vi "Format Gluing Config.vi"(4 "Active Paths":T2=[FALSE, FALSE, FALSE, FALSE], 6 "Glue Pathways":T3=[{"HDI Slot "=0, "Stamp Slot"=0, "Glue Slot"=0, "Weight Slot"=0, "BBM Slot"=0}, {"HDI Slot "=1, "Stamp Slot"=1, "Glue Slot"=1, "Weight Slot"=1, "BBM Slot"=1}, {"HDI Slot "=2, "Stamp Slot"=2, "Glue Slot"=2, "Weight Slot"=2, "BBM Slot"=2}, {"HDI Slot "=3, "Stamp Slot"=3, "Glue Slot"=3, "Weight Slot"=3, "BBM Slot"=3}] {"BBM Slot" items=["Slot 1", "Slot 2", "Slot 3", "Slot 4"]; "Weight Slot" items=["Slot 1", "Slot 2", "Slot 3", "Slot 4"]; "Glue Slot" items=["Slot 1", "Slot 2", "Slot 3", "Slot 4"]; "Stamp Slot" items=["Slot 1", "Slot 2", "Slot 3", "Slot 4"]; "HDI Slot" items=["Slot 1", "Slot 2", "Slot 3", "Slot 4"]}, 8 "error in":errorcluster, 9 "Chuck Module Used for BBM:":T1 items=["Chuck 1", "Chuck 2", "Chuck 3", "Chuck 4"], 10 "Worktable":refnum<class "WorkTable Class.lvclass">, 11 "Console Log in":refnum<class "Console Log.lvclass">) -> (0 "error out":errorcluster, 2 "Formatted Worktable Config":string, 3 "Console Log out":refnum<class "Console Log.lvclass">)   [LabVIEW 2011, in "Console Log.lvclass"]
uses:
  Console Log.lvclass
  Shared Components/WorkTable Class/WorkTable Class.lvclass
  Gluing Application/UI typedefs/Glue Paths.ctl
  Gluing Application/UI typedefs/Glue Path.ctl
  Gluing Application/UI typedefs/Active Paths.ctl
  Gluing Application/UI typedefs/BBM Chuck Used.ctl
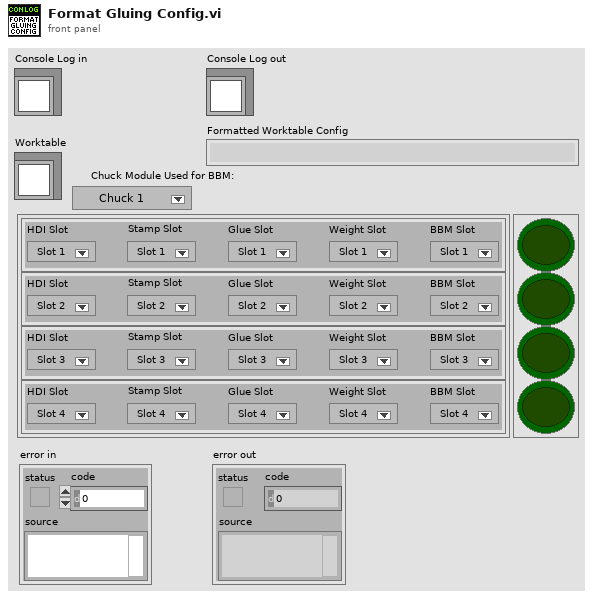
[diagram p1: front panel]
types:
  T1 = typedef "BBM Chuck Used.ctl" = i32
  T2 = typedef "Active Paths.ctl" = bool[]
  T3 = typedef "Glue Paths.ctl" = T4[]
  T4 = typedef "Glue Path.ctl" = cluster{"HDI Slot ":i32, "Stamp Slot":i32, "Glue Slot":i32, "Weight Slot":i32, "BBM Slot":i32}
  T5 = typedef "Worktable_Module Slot.ctl" = cluster{"Slot State":enum16{"Empty", "Bare HDI", "Unglued", "Stamped", "PartOnTop", "Weighted", "Unpotted", "Potted"}, "BBM Type":enum16{"None", "BBM", "GlassSlide"}, "HDI Type":enum16{"None", "HDI", "Polyimide"}, "Vacuum Channel":u8, "Location/Orientation BBM":T6, "Location/Orientation HDI":T6, "S/N":string}
  T6 = typedef "Position_Orientation.ctl" = cluster{"Center":refnum<class "Vec3d Class.lvclass">, "Orientation":refnum<class "Orient3d Class.lvclass">}
  T7 = typedef "Worktable_Stamps.ctl" = cluster{"Stamp Slots":T8[], "Vacuum Channel":i32}
  T8 = typedef "Worktable_Stamp.ctl" = cluster{"Stamp State":enum16{"Empty", "Populated", "Used"}, "Location/Orientation":T6, "Stamp Type":T9}
  T9 = typedef "Stamp Type.ctl" = enum16{"Stamp 1", "Stamp 2", "Stamp 3", "Stamp 4", "Stamp 5"}
  T10 = typedef "Worktable_Glue Reservoir.ctl" = cluster{"Glue Reservoir Slots":cluster{"Reservoir State":enum16{"Empty", "Full", "Used"}, "Center":refnum<class "Vec3d Class.lvclass">}[], "Vacuum Channel":i32}
  T11 = typedef "Worktable_Weights.ctl" = cluster{"Weight Slots":T12[], "Vacuum Channel":i32}
  T12 = typedef "Worktable_Weight.ctl" = cluster{"Weight State":enum16{"Empty", "Populated"}, "Weight Type":T13, "Location/Orientation":T6}
  T13 = typedef "Weight Type.ctl" = enum16{"Weight 1", "Weight 2", "Weight 3", "Weight 4", "Weight 5", "Weight 6", "Weight 7", "Weight 8"}
  T14 = cluster{"Reservoir State":enum16{"Empty", "Full", "Used"}, "Center":refnum<class "Vec3d Class.lvclass">}[]
  T15 = enum16{"Empty", "Bare HDI", "Unglued", "Stamped", "PartOnTop", "Weighted", "Unpotted", "Potted"}
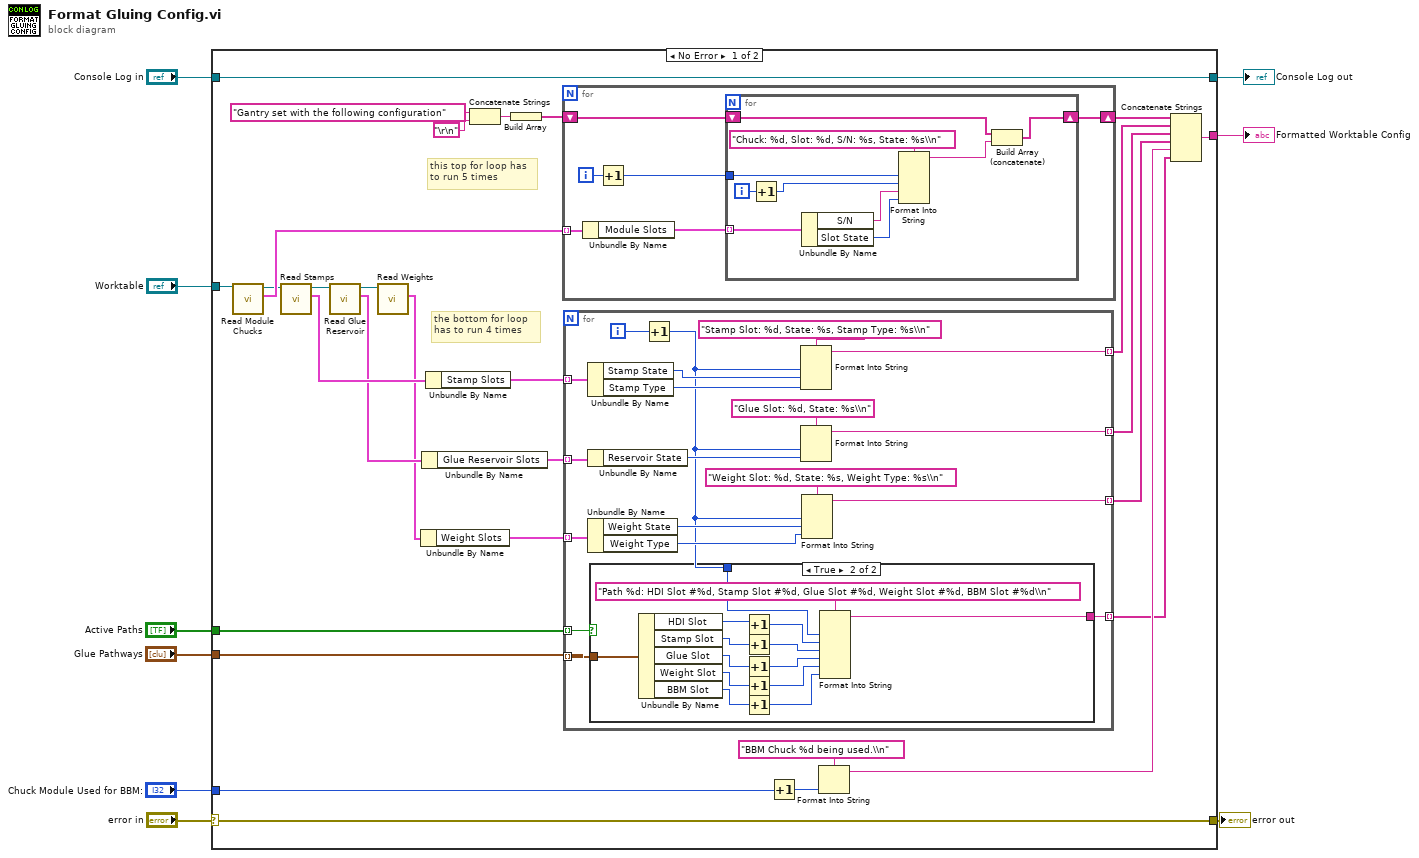
[diagram p0: block diagram]
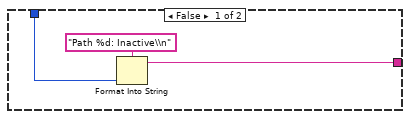
[diagram p2: hidden frame]
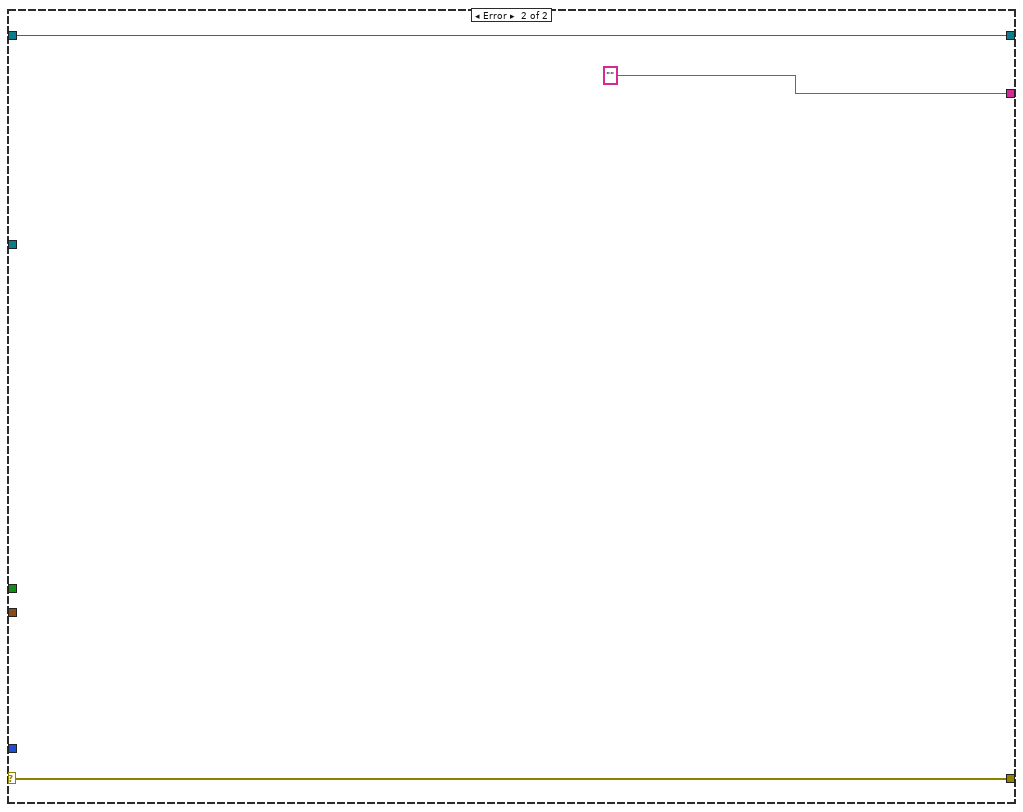
[diagram p3: hidden frame]
diagram:
  n1 = case shown="No Error" "error in" {
    selector: "error in" -> [w37 w93]
    tunnel: [w37 w93] -> w8
    tunnel: [w38 w92] -> w6
    tunnel: "Console Log in" -> [w38 w92]
    tunnel: "Worktable" -> [w29 _]
    tunnel: [w34 ""] -> w4
    tunnel: "Glue Pathways" -> [w22 _]
    tunnel: "Active Paths" -> [w21 _]
    tunnel: "Chuck Module Used for BBM:" -> [w10 _]
    frame No Error {
      # "this top for loop has\nto run 5 times"
      # "the bottom for loop\nhas to run 4 times"
      n2 = call-dynamic "Read Module Chucks.vi"("WorkTable in"=w29) -> ("Module Chucks"=w36:cluster{"Module Slots":T5[]}[], "WorkTable out"=w28:refnum<class "WorkTable Class.lvclass">)  [unwired: 8 in, 1 out]
      n3 = call-dynamic "Read Stamps.vi"("WorkTable Class in"=w28) -> ("Stamps"=w25:T7, "WorkTable Class out"=w27:refnum<class "WorkTable Class.lvclass">)  [unwired: 8 in, 1 out]
      n4 = call-dynamic "Read Glue Reservoir.vi"("WorkTable Class in"=w27) -> ("Glue Reservoir"=w24:T10, "WorkTable Class out"=w26:refnum<class "WorkTable Class.lvclass">)  [unwired: 8 in, 1 out]
      n5 = call-dynamic "Read Weights.vi"("WorkTable Class in"=w26) -> ("Weights"=w23:T11)  [unwired: 8 in, 2 out]
      n6 = Unbundle By Name(w23) -> ("Weight Slots"=w18:T12[])
      n7 = Unbundle By Name(w24) -> ("Glue Reservoir Slots"=w19:T14)
      n8 = Unbundle By Name(w25) -> ("Stamp Slots"=w20:T8[])
      n9 = Concatenate Strings("Gantry set with the following configuration", "\r\n") -> (w31:string)
      n10 = Build Array(w31) -> (w30:string[])
      n11 = for {
        tunnel: w36 -> [w80] mode=indexing
        shift-right: [w76] -> w35
        shift-left: w30 -> [w77]
        i -> [w78]
        n12 = Unbundle By Name(w80) -> ("Module Slots"=w79:T5[])
        n13 = Increment(x=w78) -> (x+1=w75:i32)
        n14 = for {
          tunnel: w79 -> [w90] mode=indexing
          tunnel: w75 -> [w88]
          shift-right: [w81] -> w76
          shift-left: w77 -> [w83]
          i -> [w89]
          n15 = Increment(x=w89) -> (x+1=w87:i32)
          n16 = Unbundle By Name(w90) -> ("S/N"=w85:string, "Slot State"=w84:T15)
          n17 = Format Into String(format string="Chuck: %d, Slot: %d, S/N: %s, State: %s\\n", w88, w87, w85, w84) -> (resulting string=w82:string)  [unwired: 2 in, 1 out]
          n18 = Build Array (concatenate)(w83, w82) -> (w81:string[])
        }
      }
      n19 = for {
        tunnel: w20 -> [w57] mode=indexing
        tunnel: w19 -> [w56] mode=indexing
        tunnel: w18 -> [w55] mode=indexing
        tunnel: [w46] -> w17 mode=indexing
        tunnel: [w45] -> w16 mode=indexing
        tunnel: [w44] -> w15 mode=indexing
        tunnel: w22 -> [w43] mode=indexing
        tunnel: w21 -> [w42] mode=indexing
        tunnel: [w41] -> w12 mode=indexing
        i -> [w40]
        n20 = Unbundle By Name(w57) -> ("Stamp State"=w53:enum16{"Empty", "Populated", "Used"}, "Stamp Type"=w52:T9)
        n21 = Unbundle By Name(w56) -> ("Reservoir State"=w50:enum16{"Empty", "Full", "Used"})
        n22 = Unbundle By Name(w55) -> ("Weight State"=w48:enum16{"Empty", "Populated"}, "Weight Type"=w47:T13)
        n23 = Increment(x=w40) -> (x+1=w39:i32)
        n24 = case shown="True" w42 {
          tunnel: w43 -> [_ w74]
          tunnel: w39 -> [w60 w73]
          tunnel: [w59 w71] -> w41
          frame False {
            n25 = Format Into String(format string="Path %d: Inactive\\n", w60) -> (resulting string=w59:string)  [unwired: 2 in, 1 out]
          }
          frame True {
            n26 = Unbundle By Name(w74) -> ("HDI Slot"=w70:i32, "Stamp Slot"=w69:i32, "Glue Slot"=w68:i32, "Weight Slot"=w67:i32, "BBM Slot"=w66:i32)
            n27 = Increment(x=w70) -> (x+1=w65:i32)
            n28 = Increment(x=w69) -> (x+1=w64:i32)
            n29 = Increment(x=w68) -> (x+1=w63:i32)
            n30 = Increment(x=w67) -> (x+1=w61:i32)
            n31 = Increment(x=w66) -> (x+1=w62:i32)
            n32 = Format Into String(format string="Path %d: HDI Slot #%d, Stamp Slot #%d, Glue Slot #%d, Weight Slot #%d, BBM Slot #%d\\n", w73, w65, w64, w63, w61, w62) -> (resulting string=w71:string)  [unwired: 2 in, 1 out]
          }
        }
        n33 = Format Into String(format string="Stamp Slot: %d, State: %s, Stamp Type: %s\\n", w39, w53, w52) -> (resulting string=w46:string)  [unwired: 2 in, 1 out]
        n34 = Format Into String(format string="Glue Slot: %d, State: %s\\n", w39, w50) -> (resulting string=w45:string)  [unwired: 2 in, 1 out]
        n35 = Format Into String(format string="Weight Slot: %d, State: %s, Weight Type: %s\\n", w39, w48, w47) -> (resulting string=w44:string)  [unwired: 2 in, 1 out]
      }
      n36 = Increment(x=w10) -> (x+1=w11:T1)
      n37 = Format Into String(format string="BBM Chuck %d being used.\\n", w11) -> (resulting string=w13:string)  [unwired: 2 in, 1 out]
      n38 = Concatenate Strings(w35, w17, w16, w15, w13, w12) -> (w34:string)
    }
    frame Error {
    }
  }
  "error out" <- w8
  "Console Log out" <- w6
  "Formatted Worktable Config" <- w4
